vi "IniEVEScrew_offset.vi"(8 "error in":errorcluster, 10 "Screw section":string="offset", 11 "INI file path":path=path "D:/ZDX201 塗膠螺絲鎖固自動化_鴻海/ZDX201_LabView/iniData/screw_iniData.ini") -> (2 "Offset array":dbl[](array[numeric]))   [LabVIEW 2019]
uses:
  <vilib>/Utility/config.llb/Read Key (Double).vi
  <vilib>/Utility/config.llb/NI_LVConfig.lvlib
panel:
  out "error out":errorcluster
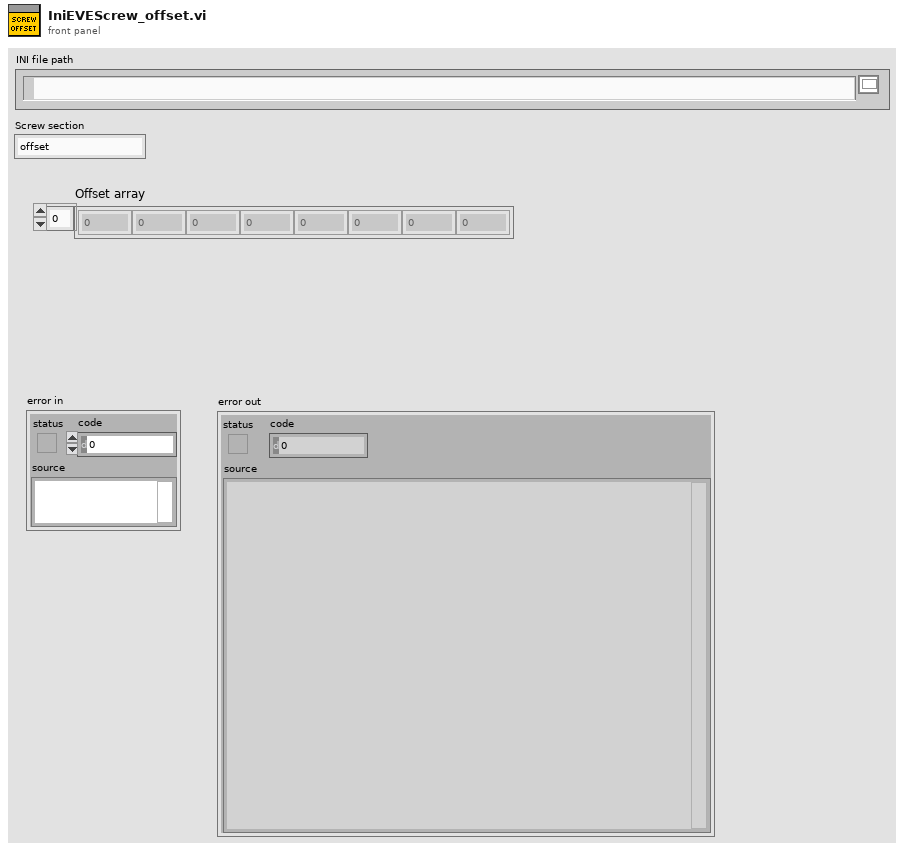
[diagram p1: front panel]
types:
  T1 = typedef "NI_LVConfig.lvlib/Config Data RefNum.ctl" = refnum<k1>
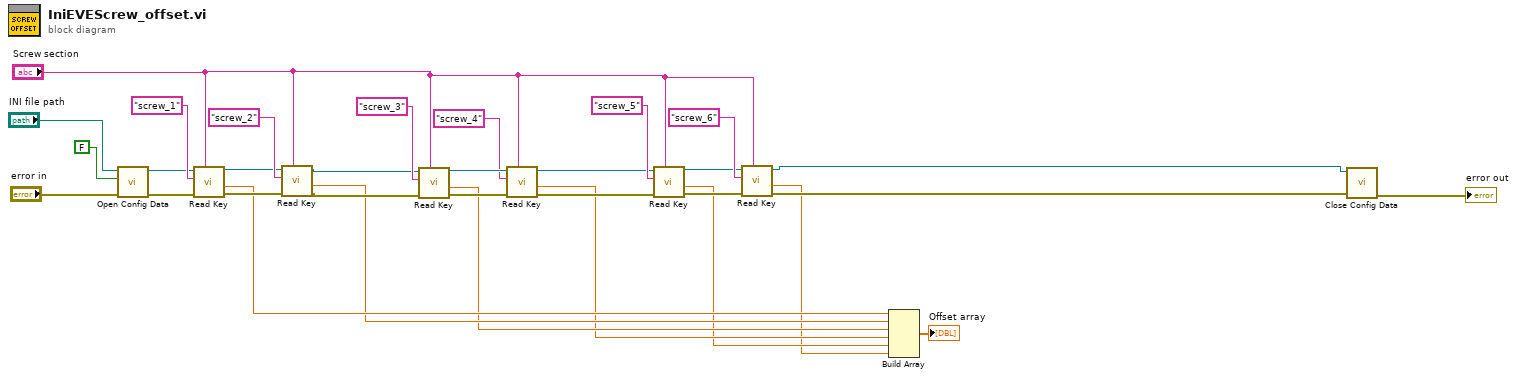
[diagram p0: block diagram]
diagram:
  n1 = call <vilib>:"Open Config Data.vi"("error in (no error)"="error in", "create file if necessary (T)"=FALSE ("create file if necessary? (T)"), "configuration file path"="INI file path") -> ("error out"=w30:errorcluster, "refnum"=w28:T1)  [unwired: 6 in, 1 out]
  n2 = call-poly <vilib>:"Read Key.vi"("section"="Screw section", "error in (no error)"=w30, "key"="screw_1", "refnum"=w28) -> ("error out"=w23:errorcluster, "value"=w7:dbl, "refnum out"=w24:T1)  [unwired: 1 in, 4 out]
  n3 = call-poly <vilib>:"Read Key.vi"("section"="Screw section", "error in (no error)"=w23, "key"="screw_2", "refnum"=w24) -> ("error out"=w13:errorcluster, "value"=w6:dbl, "refnum out"=w14:T1)  [unwired: 1 in, 4 out]
  n4 = call-poly <vilib>:"Read Key.vi"("section"="Screw section", "error in (no error)"=w13, "key"="screw_3", "refnum"=w14) -> ("error out"=w22:errorcluster, "value"=w5:dbl, "refnum out"=w21:T1)  [unwired: 1 in, 4 out]
  n5 = call-poly <vilib>:"Read Key.vi"("section"="Screw section", "error in (no error)"=w22, "key"="screw_4", "refnum"=w21) -> ("error out"=w11:errorcluster, "value"=w4:dbl, "refnum out"=w12:T1)  [unwired: 1 in, 4 out]
  n6 = call-poly <vilib>:"Read Key.vi"("section"="Screw section", "error in (no error)"=w11, "key"="screw_5", "refnum"=w12) -> ("error out"=w15:errorcluster, "value"=w3:dbl, "refnum out"=w16:T1)  [unwired: 1 in, 4 out]
  n7 = call-poly <vilib>:"Read Key.vi"("section"="Screw section", "error in (no error)"=w15, "key"="screw_6", "refnum"=w16) -> ("error out"=w8:errorcluster, "value"=w2:dbl, "refnum out"=w9:T1)  [unwired: 1 in, 4 out]
  n8 = Build Array(w7, w6, w5, w4, w3, w2) -> (→"Offset array":dbl[])
  n9 = call <vilib>:"Close Config Data.vi"("error in (no error)"=w8, "refnum"=w9) -> ("error out"=→"error out":errorcluster)  [unwired: 1 in, 8 out]
